vi "Create Preset commands From Position Position-Power Row.vi"(10 "Create SlowZ commands_Enum":T1, 11 "Position-Power Row":dbl[](array[numeric])) -> (3 "concatenated string":string)   [LabVIEW 2012]
doc: "SciScan 1.2 160622"
uses:
  Create Preset commands ENUM.ctl
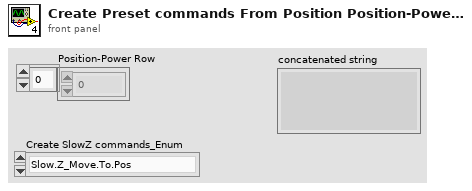
[diagram p1: front panel]
types:
  T1 = typedef "Create Preset commands ENUM.ctl" = enum16{"Slow.Z_Move.To.Pos", "Slow.Z_Laser.Power", "Slow.Z_Record", "Tiling_Move.To.Pos", "Tiling_Laser.Power", "Tiling_Record"}
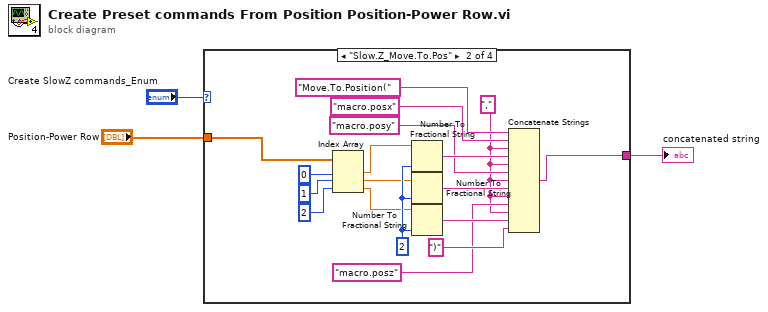
[diagram p0: block diagram]
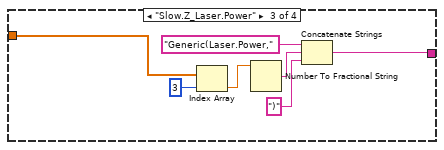
[diagram p3: hidden frame]
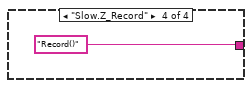
[diagram p4: hidden frame]
diagram:
  n1 = case shown="\"Slow.Z_Move.To.Pos\"" "Create SlowZ commands_Enum" {
    tunnel: [_ w21 w23 "Record()" ("Variable Name in")] -> w3
    tunnel: "Position-Power Row" -> [_ w11 w24 _]
    frame Default {
    }
    frame "Slow.Z_Move.To.Pos" {
      w20 = i16 2 ("precision (6)")
      w4 = "," ("Variable Name in")
      n2 = Index Array(array=w11, index #1=0 ("index (row)"), index #2=1 ("index (row)"), index #3=2 ("index (row)")) -> (element #1=w12:dbl, element #2=w13:dbl, element #3=w14:dbl)
      n3 = Number To Fractional String(number=w12, precision (6)=w20) -> (F-format string=w16:string)  [unwired: 2 in]
      n4 = Number To Fractional String(number=w13, precision (6)=w20) -> (F-format string=w17:string)  [unwired: 2 in]
      n5 = Number To Fractional String(number=w14, precision (6)=w20) -> (F-format string=w18:string)  [unwired: 2 in]
      n6 = Concatenate Strings("Move.To.Position(" ("Variable Name in"), "macro.posx" ("Variable Name in"), w4, w16, w4, "macro.posy" ("Variable Name in"), w4, w17, w4, "macro.posz" ("Variable Name in"), w4, w18, ")" ("Variable Name in")) -> (w21:string)
    }
    frame "Slow.Z_Laser.Power" {
      n7 = Index Array(array=w24, index=3 ("disabled index (col)")) -> (element=w27:dbl)
      n8 = Number To Fractional String(number=w27) -> (F-format string=w26:string)  [unwired: 3 in]
      n9 = Concatenate Strings("Generic(Laser.Power," ("Variable Name in"), w26, ")" ("string")) -> (w23:string)
    }
    frame "Slow.Z_Record" {
    }
  }
  "concatenated string" <- w3
